vi "From Mapped Strings.vi"(0 "Strings":string[](array[string]), 1 "Key":string) -> (2 "Array":refnum<class "Array.lvclass">)   [LabVIEW 2018, in "Toolkit.lvlib" / "Types.lvlib" / "Array.lvclass"]
uses:
  Array.lvclass
  Array.lvclass/Array.ctl
  Map/Map.lvclass
  D:/Users/cfield/Code/Field R&D Services/Mustache/LabVIEW/trunk/src/Toolkit/Data/Abstract/Abstract.lvclass
  Map/Support/From String.vi
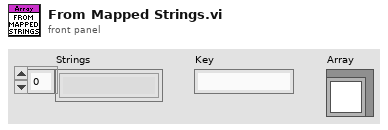
[diagram p1: front panel]
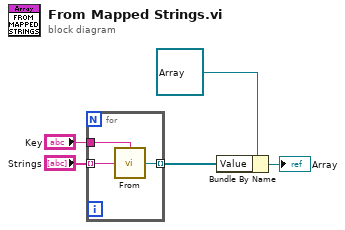
[diagram p0: block diagram]
diagram:
  n1 = for {
    tunnel: "Strings" -> [w8] mode=indexing
    tunnel: "Key" -> [w7]
    tunnel: [w6] -> w1 mode=indexing
    n2 = call-poly "From.vi"("Value"=w8, "Key"=w7) -> ("Map"=w6:refnum<class "Map.lvclass">)
  }
  n3 = Bundle By Name(cluster=refnum<class "Array.lvclass"> refnum ("Toolkit.lvlib:Data.lvlib:Array.lvclass"), "Value"=w1) -> (→"Array":refnum<class "Array.lvclass">)
